vi "Polling Core.vi"(8 "Error In":errorcluster, 11 "CS++Nanotec in":refnum<class "CS++Nanotec.lvclass">) -> (0 "Error Out":errorcluster, 3 "CS++Nanotec out":refnum<class "CS++Nanotec.lvclass">)   [LabVIEW 2015, in "CS++Nanotec.lvlib" / "CS++Nanotec.lvclass"]
uses:
  CS++Nanotec.lvclass
  CSPP_Core/Actors/CS++BaseActor/CS++BaseActor.lvclass/CS++BaseActor.ctl
  CSPP_Core/Actors/CS++BaseActor/CS++BaseActor.lvclass
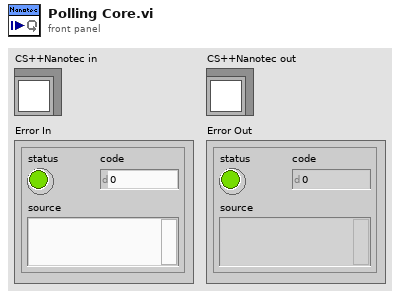
[diagram p1: front panel]
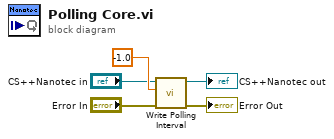
[diagram p0: block diagram]
diagram:
  n1 = call "Write Polling Interval.vi"("error in (no error)"="Error In", "Polling Interval"=dbl[unit] -1.0, "CS++BaseActor in"="CS++Nanotec in") -> ("error out"=→"Error Out":errorcluster, "CS++BaseActor out"=→"CS++Nanotec out":refnum<class "CS++Nanotec.lvclass">)  [unwired: 7 in]
